vi "MCListbox Event - Sort Table (Array Selection).vi"(9 "Clicked Color":u32(colorbox), 10 "Sort Order Boolean Ref":refnum<vi>, 11 "MCListBox Ref":refnum<vi>) -> (3 "ItemNames":string[][](array[string]))   [LabVIEW 2013]
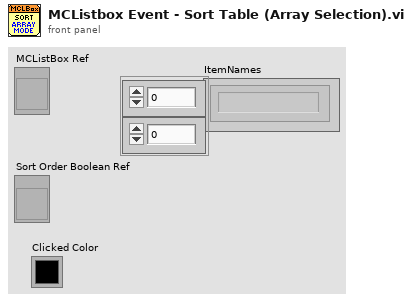
[diagram p1: front panel]
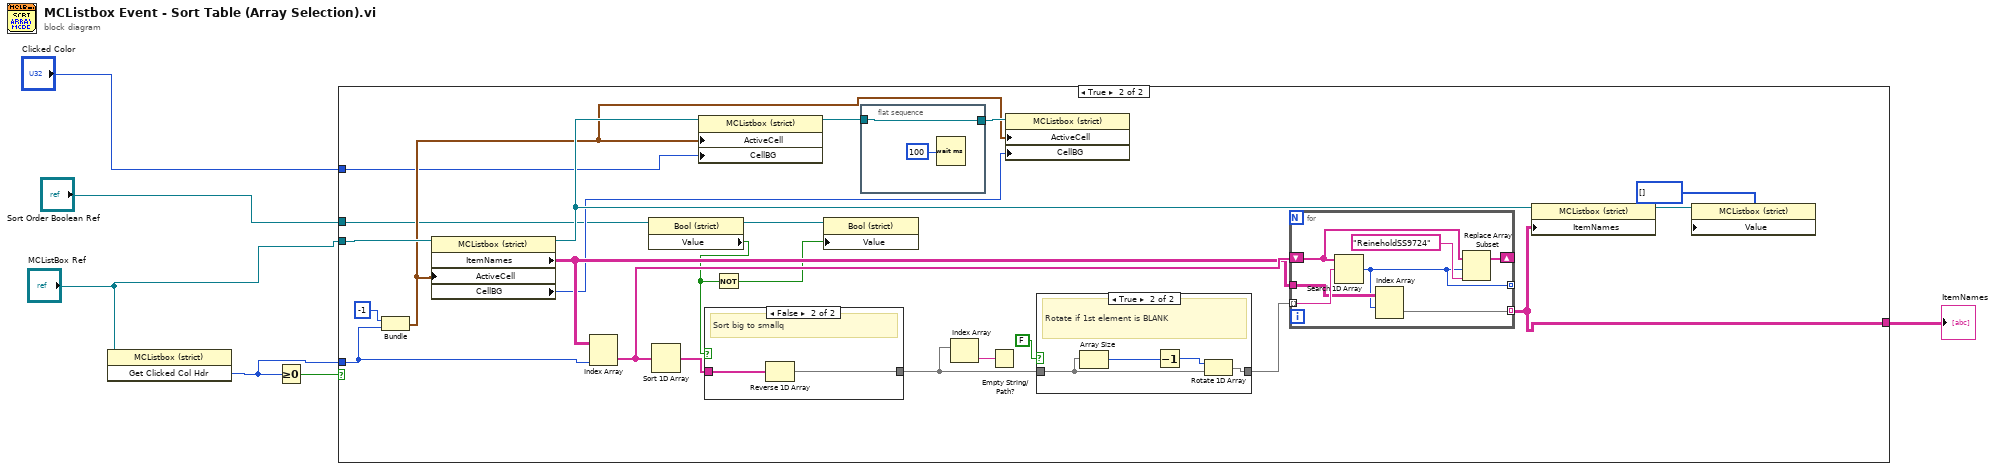
[diagram p0: block diagram]
diagram:
  n1 = invoke class="MCListbox (strict)" method="Get Clicked Col Hdr"(reference="MCListBox Ref") -> ("Get Clicked Column Header"=w2:i32)  [unwired: 2 in, 2 out]
  n2 = Greater Or Equal To 0?(x=w2) -> (x >= 0?=w1:bool)
  n3 = case shown="True" w1 {
    tunnel: "MCListBox Ref" -> [_ w23]
    tunnel: w2 -> [_ w18]
    tunnel: [_ w12] -> w4
    tunnel: "Clicked Color" -> [_ w11]
    tunnel: "Sort Order Boolean Ref" -> [_ w10]
    frame False {
    }
    frame True {
      n4 = Bundle(-1, "Get Clicked Column Header"=w18) -> (w15:cluster{i32, "Get Clicked Column Header":i32})  [unwired: 1 in]
      n5 = property class="MCListbox (strict)"(reference=w23, "ActiveCell"=w15) -> (reference out=w20:refnum<vi>, "ItemNames"=w22:string[][], "CellBG"=w14:u32)  [unwired: 1 in, 1 out]
      n6 = Index Array(array=w22, index (col)=w18) -> (element=w26:string[])  [unwired: 1 in]
      n7 = property class="Bool (strict)"(reference=w10) -> (reference out=w9:refnum<vi>, "Value"=w8:bool)  [unwired: 1 in, 1 out]
      n8 = Sort 1D Array(array=w26) -> (sorted array=w29:string[])
      n9 = property class="MCListbox (strict)"(reference=w20, "ActiveCell"=w15, "CellBG"=w11) -> (reference out=w17:refnum<vi>)  [unwired: 1 in, 1 out]
      n10 = case shown="False" w8 {
        tunnel: w29 -> [w37 w39]
        tunnel: [w37 w38] -> w24
        frame True {
          # "Sort small to big p"
        }
        frame False {
          # "Sort big to smallq"
          n11 = Reverse 1D Array(array=w39) -> (reversed array=w38:string[])
        }
      }
      n12 = Not(x=w8) -> (.not. x?=w7:bool)
      n13 = property class="Bool (strict)"(reference=w9, "Value"=w7) -> ()  [unwired: 1 in, 2 out]
      n14 = flat-sequence {
        tunnel: w17 -> [w31]
        tunnel: [w31] -> w16
        frame #0 {
          n15 = Wait (ms)(milliseconds to wait=u32 100) -> ()  [unwired: 1 out]
        }
      }
      n16 = Index Array(array=w24) -> (element=w25:string)  [unwired: 1 in]
      n17 = Empty String/Path?(string/path=w25) -> ()  [unwired: 1 out]
      n18 = property class="MCListbox (strict)"(reference=w16, "ActiveCell"=w15, "CellBG"=w14) -> ()  [unwired: 1 in, 2 out]
      n19 = case shown="True" FALSE {
        tunnel: w24 -> [w32 w35]
        tunnel: [w32 w36] -> w21
        frame False {
        }
        frame True {
          # "Rotate if 1st element is BLANK"
          n20 = Array Size(array=w35) -> (size(s)=w34:i32)
          n21 = Decrement(x=w34) -> (x-1=w33:i32)
          n22 = Rotate 1D Array(1:w35, 2:w33) -> (0:w36:string[])
        }
      }
      n23 = for {
        tunnel: w21 -> [w46] mode=indexing
        shift-right: [w43] -> _
        shift-left: w26 -> [w45]
        tunnel: [w40] -> _ mode=indexing
        tunnel: w22 -> [w42]
        tunnel: [w41] -> w12 mode=indexing
        n24 = Search 1D Array(1D array=w45, element=w46) -> (index of element=w40:i32)  [unwired: 1 in]
        n25 = Index Array(array=w42, index (row)=w40) -> (element=w41:string[])  [unwired: 1 in]
        n26 = Replace Array Subset(array=w45, new element="ReineholdSS9724" ("new element/subarray"), index=w40) -> (w43:string[])
      }
      n27 = property class="MCListbox (strict)"(reference=w20, "ItemNames"=w12) -> (reference out=w28:refnum<vi>)  [unwired: 1 in, 1 out]
      n28 = property class="MCListbox (strict)"(reference=w28, "Value"=i32[] []) -> ()  [unwired: 1 in, 2 out]
    }
  }
  "ItemNames" <- w4
